vi "labor.vi"() -> ()   [LabVIEW 2010]
panel:
  in  "neuer Wert":i32
  in  "Stopp":bool
  out "Wert":i32
  in  "Wert ändern":bool
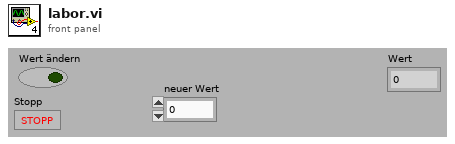
[diagram p1: front panel]
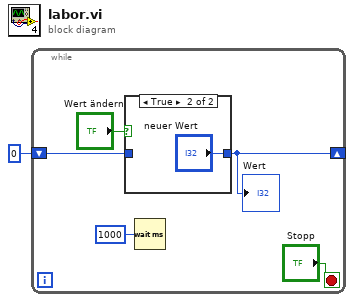
[diagram p0: block diagram]
diagram:
  n1 = while {
    shift-right: [w3] -> _
    shift-left: 0 -> [w4]
    stop <- "Stopp" stop-if-true
    n2 = case shown="True" "Wert ändern" {
      tunnel: w4 -> [w7 _]
      tunnel: [w7 "neuer Wert"] -> w3
      frame False {
      }
      frame True {
      }
    }
    "Wert" <- w3
    n3 = Wait (ms)(milliseconds to wait=u32 1000 ("Zu wartende ms")) -> ()  [unwired: 1 out]
  }
